vi "MultiChannel Moving Average Filter PtByPt.vi"(7 "Initialize":bool, 10 "Number of Averages":u32=100, 11 "X":dbl[](array[numeric])) -> (3 "Filtered X":dbl[](array[numeric]))   [LabVIEW 2011, in "Filter VIs.lvlib"]
uses:
  Filter VIs.lvlib
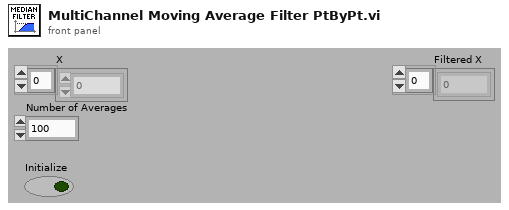
[diagram p1: front panel]
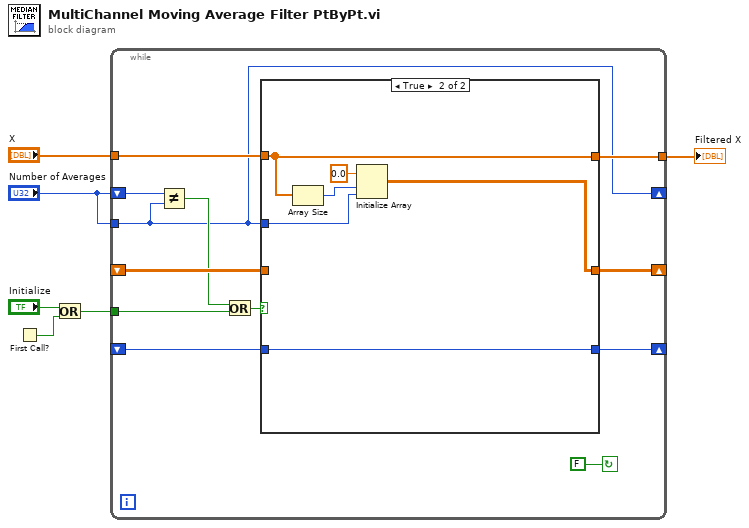
[diagram p0: block diagram]
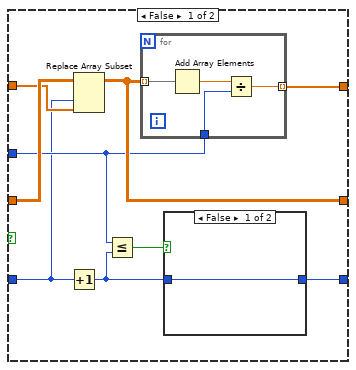
[diagram p2: hidden frame]
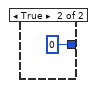
[diagram p3: hidden frame]
diagram:
  n1 = First Call?() -> (First Call?: T/F=w2:bool)
  n2 = Or(x="Initialize", y=w2) -> (x .or. y?=w3:bool)
  n3 = while {
    tunnel: w3 -> [w11]
    tunnel: "X" -> [w18]
    shift-right: [w16] -> _
    shift-left: _ -> [w15]
    tunnel: [w14] -> w5
    shift-right: [w12] -> _
    shift-left: _ -> [w13]
    shift-right: [w7] -> _
    shift-left: "Number of Averages" -> [w9]
    tunnel: "Number of Averages" -> [w7]
    stop <- FALSE continue-if-true
    n4 = Not Equal?(x=w9, y=w7) -> (x != y?=w8:bool)
    n5 = Or(x=w8, y=w11) -> (x .or. y?=w10:bool)
    n6 = case shown="True" w10 {
      tunnel: w18 -> [w26 w35]
      tunnel: w7 -> [w22 w37]
      tunnel: [w24 w34] -> w16
      tunnel: w15 -> [w27 _]
      tunnel: [w25 w35] -> w14
      tunnel: w13 -> [w19 w36]
      tunnel: [w23 w36] -> w12
      frame False {
        n7 = Increment(x=w19) -> (x+1=w20:i32)
        n8 = Replace Array Subset(array=w27, new element=w26, index (col)=w19) -> (w24:dbl[][])  [unwired: 1 in]
        n9 = Less Or Equal?(x=w22, y=w20) -> (x <= y?=w21:bool)
        n10 = for {
          tunnel: w24 -> [w33] mode=indexing
          tunnel: w22 -> [w31]
          tunnel: [w30] -> w25 mode=indexing
          n11 = Add Array Elements(numeric array=w33) -> (sum=w32:dbl)
          n12 = Divide(x=w32, y=w31) -> (x/y=w30:dbl)
        }
        n13 = case shown="False" w21 {
          tunnel: [w28 0] -> w23
          tunnel: w20 -> [w28 _]
          frame False {
          }
          frame True {
          }
        }
      }
      frame True {
        n14 = Array Size(array=w35) -> (size(s)=w38:i32)
        n15 = Initialize Array(0.0 ("element"), w38, w37) -> (w34:dbl[][])
      }
    }
  }
  "Filtered X" <- w5
